vi "Test FDM Convert.vi"() -> ()   [LabVIEW 2010]
uses:
  FGNetFDM.ctl
  Flight Gear Data Custom Device.lvlib
panel:
  out "Cluster 2":T1={"Version"={"version"=20, "pad"=0}, "Positions"={"Doubles"={"longitude"=0.0, "latitude"=0.0, "altitude"=0.0}, "Singles"={"agl"=0.0, "phi"=0.0, "theta"=0.0, "psi"=0.0, "alpha"=0.0, "beta"=0.0}}, "Velocities"={"phidot"=0.0, "thetadot"=0.0, "psidot"=0.0, "vcas"=0.0, "climb_rate"=0.0, "v_north"=0.0, "v_east"=0.0, "v_down"=0.0, "v_wind_body_north"=0.0, "v_wind_body_east"=0.0, "v_wind_body_down"=0.0}, "Accelerations"={"A_X_pilot"=0.0, "A_Y_pilot"=0.0, "A_Z_pilot"=0.0}, "Stall"={"stall_warning"=0.0, "slip_deg"=0.0}, "Engine Status"={"num_engines"=0, "eng_state"=[0, 0, 0, 0], "rpm"=[0.0, 0.0, 0.0, 0.0], "fuel_flow"=[0.0, 0.0, 0.0, 0.0], "fuel_px"=[0.0, 0.0, 0.0, 0.0], "egt"=[0.0, 0.0, 0.0, 0.0], "cht"=[0.0, 0.0, 0.0, 0.0], "mp_osi"=[0.0, 0.0, 0.0, 0.0], "tit"=[0.0, 0.0, 0.0, 0.0], "oil_temp"=[0.0, 0.0, 0.0, 0.0], "oil_px"=[0.0, 0.0, 0.0, 0.0]}, "Consumables"={"num_tanks"=0, "fuel_quantity"=[0.0, 0.0, 0.0, 0.0]}, "Gear Status"={"num_wheels"=0, "wow"=[0, 0, 0, 0], "gear_pos"=[0.0, 0.0, 0.0, 0.0], "gear_steer"=[0.0, 0.0, 0.0, 0.0], "gear_compression"=[0.0, 0.0, 0.0, 0.0]}, "Environment"={"curr_time"=0, "warp"=0, "visibility"=0.0}, "Control Surface Positions"={"elevator"=0.0, "elevator_trim_tab"=0.0, "left_flap"=0.0, "right_flap"=0.0, "left aileron"=0.0, "right_aileron"=0.0, "rudder"=0.0, "nose_wheel"=0.0, "speedbrake"=0.0, "spoilers"=0.0}}
  in  "Cluster":T1={"Version"={"version"=20, "pad"=0}, "Positions"={"Doubles"={"longitude"=0.0, "latitude"=0.0, "altitude"=0.0}, "Singles"={"agl"=0.0, "phi"=0.0, "theta"=0.0, "psi"=0.0, "alpha"=0.0, "beta"=0.0}}, "Velocities"={"phidot"=0.0, "thetadot"=0.0, "psidot"=0.0, "vcas"=0.0, "climb_rate"=0.0, "v_north"=0.0, "v_east"=0.0, "v_down"=0.0, "v_wind_body_north"=0.0, "v_wind_body_east"=0.0, "v_wind_body_down"=0.0}, "Accelerations"={"A_X_pilot"=0.0, "A_Y_pilot"=0.0, "A_Z_pilot"=0.0}, "Stall"={"stall_warning"=0.0, "slip_deg"=0.0}, "Engine Status"={"num_engines"=0, "eng_state"=[0, 0, 0, 0], "rpm"=[0.0, 0.0, 0.0, 0.0], "fuel_flow"=[0.0, 0.0, 0.0, 0.0], "fuel_px"=[0.0, 0.0, 0.0, 0.0], "egt"=[0.0, 0.0, 0.0, 0.0], "cht"=[0.0, 0.0, 0.0, 0.0], "mp_osi"=[0.0, 0.0, 0.0, 0.0], "tit"=[0.0, 0.0, 0.0, 0.0], "oil_temp"=[0.0, 0.0, 0.0, 0.0], "oil_px"=[0.0, 0.0, 0.0, 0.0]}, "Consumables"={"num_tanks"=0, "fuel_quantity"=[0.0, 0.0, 0.0, 0.0]}, "Gear Status"={"num_wheels"=0, "wow"=[0, 0, 0, 0], "gear_pos"=[0.0, 0.0, 0.0, 0.0], "gear_steer"=[0.0, 0.0, 0.0, 0.0], "gear_compression"=[0.0, 0.0, 0.0, 0.0]}, "Environment"={"curr_time"=0, "warp"=0, "visibility"=0.0}, "Control Surface Positions"={"elevator"=0.0, "elevator_trim_tab"=0.0, "left_flap"=0.0, "right_flap"=0.0, "left aileron"=0.0, "right_aileron"=0.0, "rudder"=0.0, "nose_wheel"=0.0, "speedbrake"=0.0, "spoilers"=0.0}}
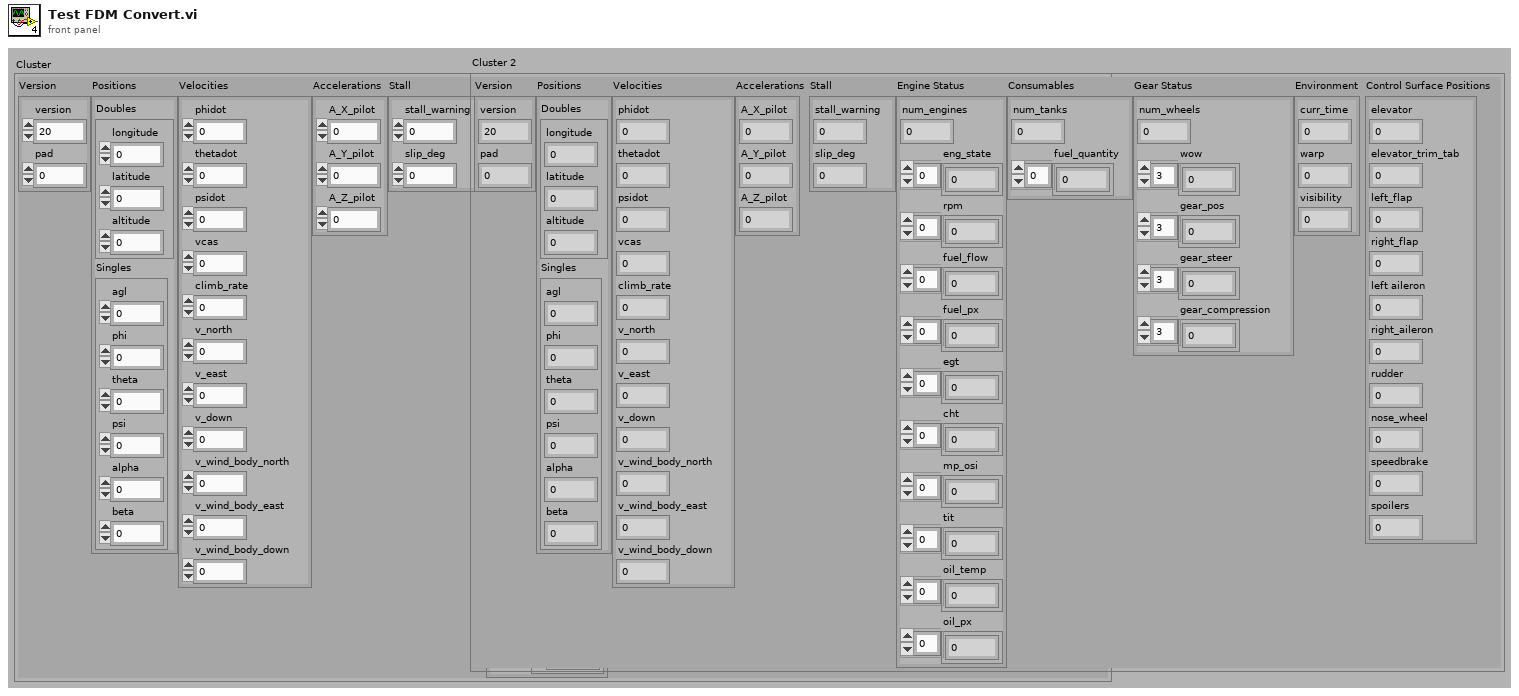
[diagram p1: front panel]
types:
  T1 = typedef "Flight Gear Data Custom Device.lvlib/FGNetFDM.ctl" = cluster{"Version":cluster{"version":u32, "pad":u32}, "Positions":cluster{"Doubles":cluster{"longitude":dbl, "latitude":dbl, "altitude":dbl}, "Singles":cluster{"agl":sgl, "phi":sgl, "theta":sgl, "psi":sgl, "alpha":sgl, "beta":sgl}}, "Velocities":cluster{"phidot":sgl, "thetadot":sgl, "psidot":sgl, "vcas":sgl, "climb_rate":sgl, "v_north":sgl, "v_east":sgl, "v_down":sgl, "v_wind_body_north":sgl, "v_wind_body_east":sgl, "v_wind_body_down":sgl}, "Accelerations":cluster{"A_X_pilot":sgl, "A_Y_pilot":sgl, "A_Z_pilot":sgl}, "Stall":cluster{"stall_warning":sgl, "slip_deg":sgl}, "Engine Status":cluster{"num_engines":u32, "eng_state":u32[], "rpm":sgl[], "fuel_flow":sgl[], "fuel_px":sgl[], "egt":sgl[], "cht":sgl[], "mp_osi":sgl[], "tit":sgl[], "oil_temp":sgl[], "oil_px":sgl[]}, "Consumables":cluster{"num_tanks":u32, "fuel_quantity":sgl[]}, "Gear Status":cluster{"num_wheels":u32, "wow":u32[], "gear_pos":sgl[], "gear_steer":sgl[], "gear_compression":sgl[]}, "Environment":cluster{"curr_time":u32, "warp":i32, "visibility":sgl}, "Control Surface Positions":cluster{"elevator":sgl, "elevator_trim_tab":sgl, "left_flap":sgl, "right_flap":sgl, "left aileron":sgl, "right_aileron":sgl, "rudder":sgl, "nose_wheel":sgl, "speedbrake":sgl, "spoilers":sgl}}
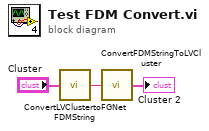
[diagram p0: block diagram]
diagram:
  n1 = call "ConvertLVClustertoFGNetFDMString.vi"("Cluster"="Cluster") -> ("FGNetFDM"=w2:string)
  n2 = call "ConvertFDMStringToLVCluster.vi"("FGNetFDM"=w2) -> ("Cluster"=→"Cluster 2":T1)
